vi "Write UserEventCommand.vi"(8 "error in (no error)":errorcluster caption="entrée d'erreur (pas d'erreur)", 10 "UserEventCommand":refnum<user-event>, 11 "Control en entrée":refnum<class "Control.lvclass">) -> (0 "error out":errorcluster caption="sortie d'erreur", 3 "Control en sortie":refnum<class "Control.lvclass">)   [LabVIEW 2015, in "Control.lvclass"]
uses:
  Control.lvclass
  Control.lvclass/Control.ctl
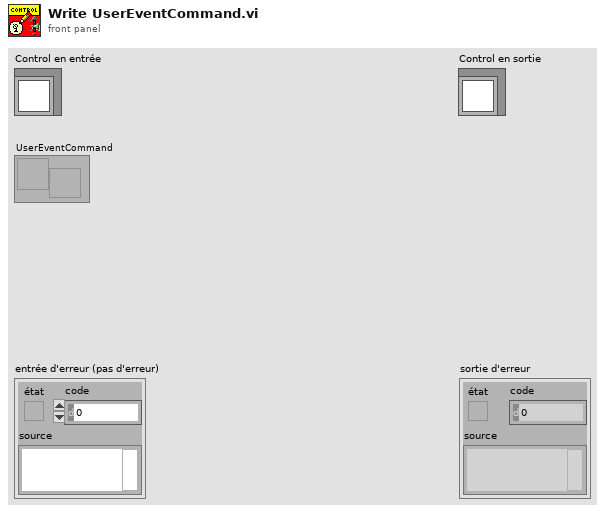
[diagram p1: front panel]
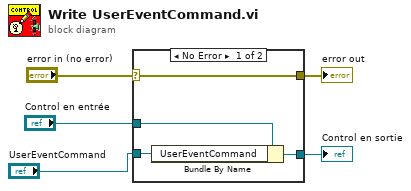
[diagram p0: block diagram]
diagram:
  n1 = case shown="No Error" "error in (no error)" {
    selector: "error in (no error)" -> [w9 w10]
    tunnel: [w9 w10] -> w4
    tunnel: [w7 w11] -> w2
    tunnel: "Control en entrée" -> [w8 w11]
    tunnel: "UserEventCommand" -> [w6 _]
    frame No Error {
      n2 = Bundle By Name(cluster=w8, "UserEventCommand"=w6) -> (w7:refnum<class "Control.lvclass">)
    }
    frame Error {
    }
  }
  "error out" <- w4
  "Control en sortie" <- w2
